vi "Get End Effector Transform.vi"(8 "error in (no error)":errorcluster, 11 "serial arm in":refnum<class "NI_Robotics_Serial Robot Arm.lvclass">) -> (0 "error out":errorcluster, 2 "end effector transform":T1, 3 "serial arm out":refnum<class "NI_Robotics_Serial Robot Arm.lvclass">)   [LabVIEW 2017, in "NI_Robotics_Serial Robot Arm.lvclass"]
doc: "Returns a homogenous transform that represents the position of the end effector of a robotic arm."
uses:
  <vilib>/robotics/Kinematics/Robot/NI_Robotics_Serial Robot Arm.lvclass
  <vilib>/Analysis/Matrix/Datatypes/RealMatrix.ctl
  <vilib>/robotics/Kinematics/Robot/NI_Robotics_Serial Robot Arm.lvclass/NI_Robotics_Serial Robot Arm.ctl
  <vilib>/Analysis/Matrix/NI_Matrix.lvlib
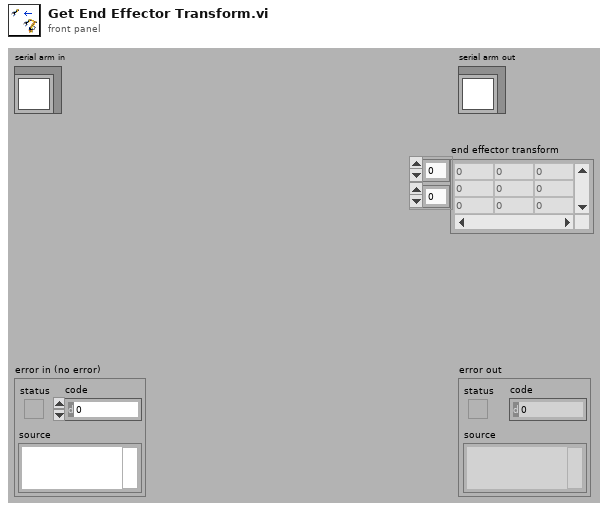
[diagram p1: front panel]
types:
  T1 = typedef "NI_Matrix.lvlib/RealMatrix.ctl" = dbl[][]
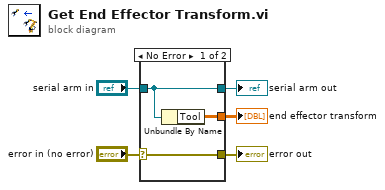
[diagram p0: block diagram]
diagram:
  n1 = case shown="No Error" "error in (no error)" {
    selector: "error in (no error)" -> [w8 w9]
    tunnel: [w8 w9] -> w4
    tunnel: [w7 w10] -> w2
    tunnel: "serial arm in" -> [w7 w10]
    tunnel: [w6 _] -> w1
    frame No Error {
      n2 = Unbundle By Name(w7) -> ("Tool"=w6:T1)
    }
    frame Error {
    }
  }
  "error out" <- w4
  "serial arm out" <- w2
  "end effector transform" <- w1
